vi "PlaMoS_RunCurrStep.vi"(8 "error in (no error)":errorcluster, 9 "Curr Iter Params":T1, 10 "StepParams":T2, 11 "FPGA VI Reference In":refnum<k20>) -> (0 "error out":errorcluster, 2 "Step Completed?":bool, 3 "FPGA VI Reference Out":refnum<k20>)   [LabVIEW 2020, in "PlannedMotionSequence.lvlib"]
doc: "Generate the Z or U reference for next iteration and updates parameters in FPGA."
uses:
  PlannedMotionSequence.lvlib
  TypeDefs/StepParams.ctl
  TypeDefs/CtrlEff Params.ctl
  TypeDefs/PosCtrl Params.ctl
  TypeDefs/HoldStateParams.ctl
  TypeDefs/CurrIterParams.ctl
  Timing/Timing Action Engine/TimingCmd Enum.ctl
  <vilib>/Utility/error.llb/Error Cluster From Error Code.vi
  <vilib>/rvi/errors/niLvFpgaAdjustHostInterfaceError.vi
  <vilib>/rvi/interface/nirviReadWriteControl/nirviReadWriteControl.xnode
  NiFpgaLv.dll
  <vilib>/rvi/interface/Simulation/niFpgaSimulationCallBeginRW.vi
  Timing/Timing Action Engine/Timing Action Engine.lvlib
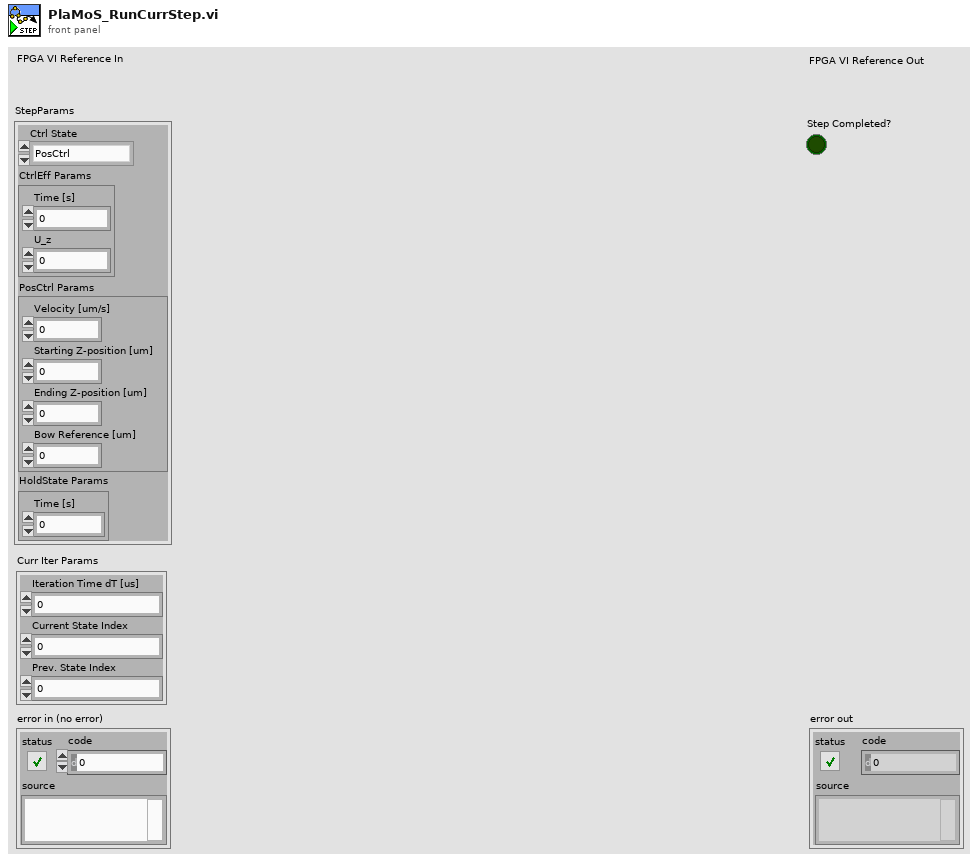
[diagram p1: front panel]
types:
  T1 = typedef "PlannedMotionSequence.lvlib/CurrIterParams.ctl" = cluster{"Iteration Time dT [us]":dbl, "Current State Index":i32, "Prev. State Index":i32}
  T2 = typedef "PlannedMotionSequence.lvlib/StepParams.ctl" = cluster{"Ctrl State":enum16{"PosCtrl", "CtrlEff", "HoldState"}, "CtrlEff Params":T3, "PosCtrl Params":T4, "HoldState Params":T5}
  T3 = typedef "PlannedMotionSequence.lvlib/CtrlEff Params.ctl" = cluster{"Time [s]":dbl, "U_z":dbl}
  T4 = typedef "PlannedMotionSequence.lvlib/PosCtrl Params.ctl" = cluster{"Velocity [um/s]":dbl, "Starting Z-position [um]":dbl, "Ending Z-position [um]":dbl, "Bow Reference [um]":dbl}
  T5 = typedef "PlannedMotionSequence.lvlib/HoldStateParams.ctl" = cluster{"Time [s]":dbl}
  T6 = typedef "Timing.lvlib/Timing Action Engine.lvlib/TimingCmd Enum.ctl" = enum16{"Reset", "Pause", "Read Time"}
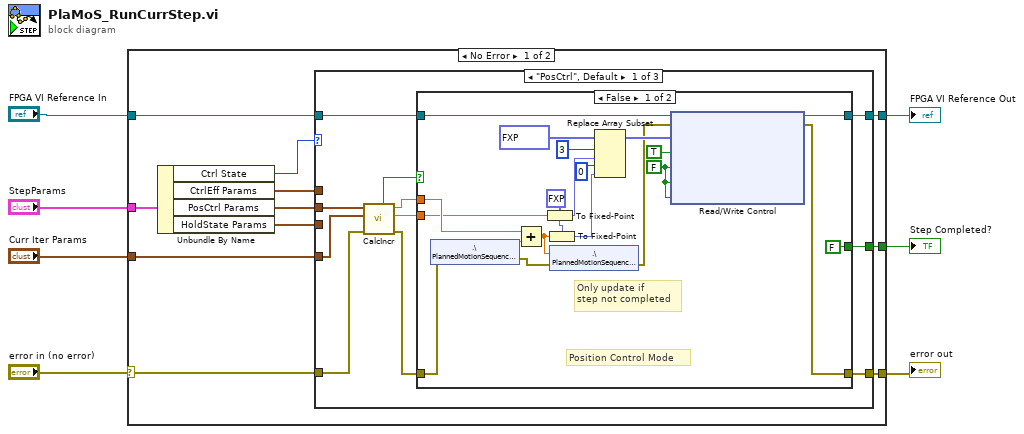
[diagram p0: block diagram]
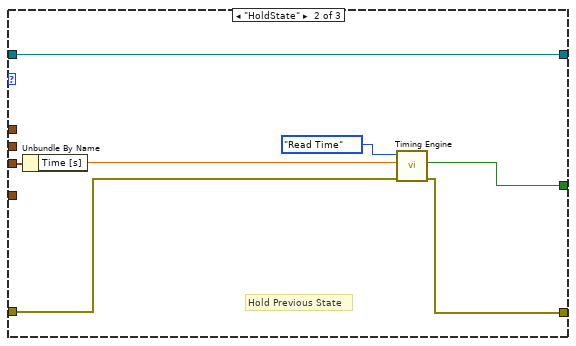
[diagram p3: hidden frame]
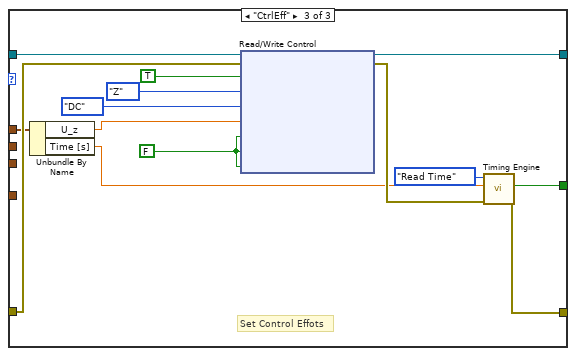
[diagram p4: hidden frame]
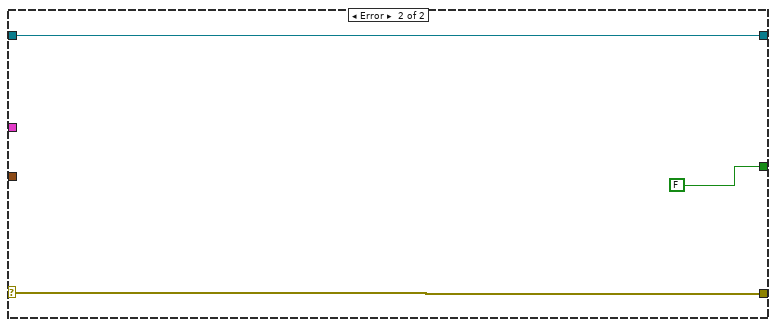
[diagram p5: hidden frame]
diagram:
  n1 = case shown="No Error" "error in (no error)" {
    selector: "error in (no error)" -> [w13 w76]
    tunnel: "StepParams" -> [w18 _]
    tunnel: "FPGA VI Reference In" -> [w16 w75]
    tunnel: [w12 w76] -> w4
    tunnel: [w11 FALSE ("Done?")] -> w3
    tunnel: [w10 w75] -> w2
    tunnel: "Curr Iter Params" -> [w9 _]
    frame No Error {
      n2 = Unbundle By Name(w18) -> ("Ctrl State"=w17:enum16{"PosCtrl", "CtrlEff", "HoldState"}, "CtrlEff Params"=w15:T3, "PosCtrl Params"=w14:T4, "HoldState Params"=w8:T5)
      n3 = case shown="\"PosCtrl\", Default" w17 {
        tunnel: w16 -> [w29 w53 w73]
        tunnel: w15 -> [_ _ w62]
        tunnel: w14 -> [w25 _ _]
        tunnel: w13 -> [w23 w56 w71]
        tunnel: [w28 w55 w69] -> w12
        tunnel: [w27 w57 w68] -> w11
        tunnel: [w26 w53 w67] -> w10
        tunnel: w9 -> [w24 _ _]
        tunnel: w8 -> [_ w59 _]
        frame "PosCtrl", Default {
          n4 = call "CalcIncr.vi"("error in (no error)"=w23, "Curr Iter Params"=w24, "PosCtrl Params"=w25) -> ("error out"=w19:errorcluster, "Bow Reference"=w21:dbl, "Incremental step"=w22:dbl, "Step Completed?"=w20:bool)  [unwired: 5 in]
          n5 = case shown="False" w20 {
            selector: w20 -> [_ w52]
            tunnel: w29 -> [w49 w51]
            tunnel: w19 -> [w33 w50]
            tunnel: [w48 w50] -> w28
            tunnel: [FALSE w52] -> w27
            tunnel: [w40 w51] -> w26
            tunnel: w22 -> [w36 _]
            tunnel: w21 -> [w35 _]
            frame False {
              w39 = fxp<+/-,25,5> 0.0 ("new element/subarray")
              w42 = FALSE ("Enable  Pos. Ref. Gen?")
              # "Position Control Mode"
              # "Only update if \nstep not completed"
              n6 = shared-variable ".\\PlannedMotionSequence.lvlib\\CurrZref"(error in=w33) -> (w34:dbl, error out=w31:errorcluster)
              n7 = Add(x=w36, y=w34) -> (x+y=w32:dbl)
              n8 = To Fixed-Point(fixed-point type=w39, number=w35) -> (fixed-point=w38:fxp<+/-,25,5>)
              n9 = To Fixed-Point(fixed-point type=w39, number=w32) -> (fixed-point=w37:fxp<+/-,25,5>)
              n10 = shared-variable ".\\PlannedMotionSequence.lvlib\\CurrZref"(w32, error in=w31) -> (error out=w30:errorcluster)
              n11 = Replace Array Subset(array=fxp<+/-,25,5>[] [0.0, 0.0, 0.0, 0.0, 0.0] ("Z,ThX,ThY,B,Bd Ref"), new element #1=w38, index #1=3 ("index"), new element #2=w37, index #2=0 ("index")) -> (w44:fxp<+/-,25,5>[])
              n12 = xnode "Read/Write Control"("FPGA VI Reference In"=w49, "error in"=w30, "Z,ThX,ThY,B,Bd Ref"=w44, "Run Controller?"=TRUE, "Enable  Pos. Ref. Gen?"=w42, "Enable  Ctrl Eff dist?"=w42, "Enable  AO dist?"=w42) -> ("FPGA VI Reference Out"=w40:refnum<k20>, "error out"=w48:errorcluster)
            }
            frame True {
            }
          }
        }
        frame "HoldState" {
          # "Hold Previous State"
          n13 = Unbundle By Name(w59) -> ("Time [s]"=w54:dbl)
          n14 = call "Timing Engine.vi"("error in (no error)"=w56, "Time Limit (sec)"=w54, "Timing Cmd In"=TimingCmd_Enum."Read Time") -> ("error out"=w55:errorcluster, "Done?"=w57:bool)  [unwired: 6 in, 1 out]
        }
        frame "CtrlEff" {
          w66 = FALSE ("Run Controller?")
          # "Set Control Effots"
          n15 = Unbundle By Name(w62) -> ("U_z"=w61:dbl, "Time [s]"=w60:dbl)
          n16 = xnode "Read/Write Control"("FPGA VI Reference In"=w73, "error in"=w71, "Enable  Ctrl Eff dist?"=TRUE, "Select CE direction"=enum8{"Z", "ThX", "ThY", "Bow", "B-d"}."Z", "CE Excitation mode"=enum8{"DC", "Sine", "Square", "WhiteNoise"}."DC", "CE Amplitude [V]"=w61, "Run Controller?"=w66, "Enable  AO dist?"=w66, "Enable  Pos. Ref. Gen?"=w66) -> ("FPGA VI Reference Out"=w67:refnum<k20>, "error out"=w70:errorcluster)
          n17 = call "Timing Engine.vi"("error in (no error)"=w70, "Time Limit (sec)"=w60, "Timing Cmd In"=TimingCmd_Enum."Read Time") -> ("error out"=w69:errorcluster, "Done?"=w68:bool)  [unwired: 6 in, 1 out]
        }
      }
    }
    frame Error {
    }
  }
  "error out" <- w4
  "FPGA VI Reference Out" <- w2
  "Step Completed?" <- w3
